vi "Get Class Referernce.vi"(8 "error in (no error)":errorcluster, 10 "ClassName":string, 11 "Application in":refnum<class "Application.lvclass">) -> (0 "error out":errorcluster, 3 "Application out":refnum<class "Application.lvclass">)   [LabVIEW 2019, in "Application.lvclass"]
doc: "Developed by Kevin Thompson\nkevin@thompsonengineering.net\n\nCopyright 2020\nThompson Engineering, LLC"
uses:
  Application.lvclass
panel:
  out "LabVIEW Object":refnum<class>
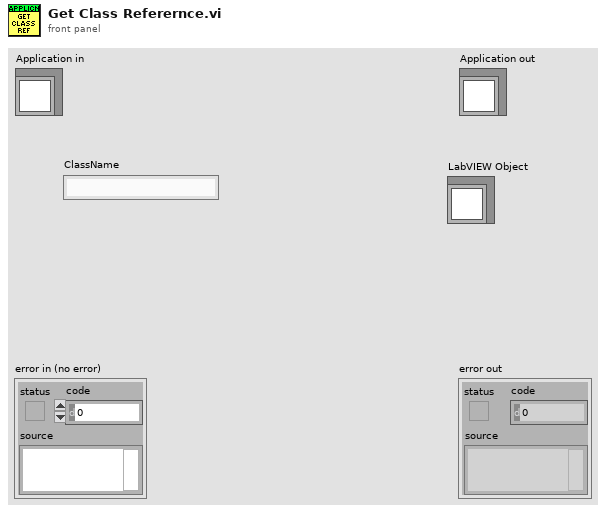
[diagram p1: front panel]
types:
  T1 = typedef "Application.lvclass/ObjData--cluster.ctl" = cluster{"Settings":T2, "Public Events":T3, "Dependency":T4, "ReadData-placeholder":T5, "VISA-placeholder":refnum<visa-resource-name>, "Subsys ClassRefs Dict":T6, "InverterWaveformsQ":T7, "RawDaqDataQ":T8}
  T2 = typedef "Application.lvclass/Settings--cluster.ctl" = cluster{"Simulation":bool}
  T3 = typedef "Application.lvclass/Public Events--cluster.ctl" = cluster{"Application.AsyncCmd Event":refnum<user-event>, "Application.AsyncMsg Event":refnum<user-event>, "stop process":refnum<user-event>}
  T4 = typedef "Application.lvclass/Dependency--cluster.ctl" = cluster{"Config":refnum<class "Config.lvclass">, "Main":refnum<class "Main.lvclass">, "ErrorHandler":refnum<class "ErrorHandler.lvclass">, "DAQ_Engine":refnum<class "DAQ_Engine.lvclass">, "Log_Engine":refnum<class "Log_Engine.lvclass">}
  T5 = typedef "Application.lvclass/Read Data--cluster.ctl" = cluster{"Data":dbl}
  T6 = typedef "TD Dynamic CVT DVR--ref.ctl" = refnum<data-value>
  T7 = typedef "InverterWaveforms--QRef.ctl" = refnum<queue>
  T8 = typedef "RawDAQDataQRef--cluster.ctl" = refnum<queue>
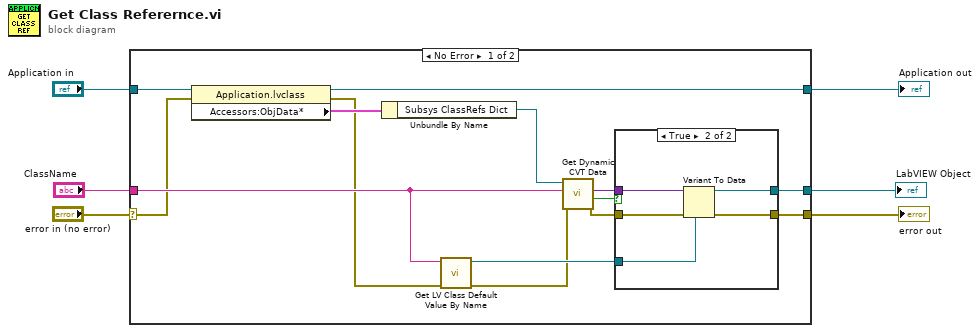
[diagram p0: block diagram]
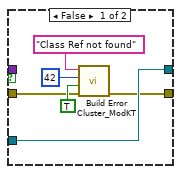
[diagram p2: hidden frame]
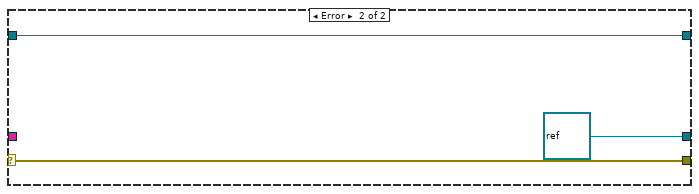
[diagram p3: hidden frame]
diagram:
  n1 = case shown="No Error" "error in (no error)" {
    selector: "error in (no error)" -> [w12 w34]
    tunnel: [w9 w34] -> w5
    tunnel: [w19 w33] -> w3
    tunnel: "Application in" -> [w20 w33]
    tunnel: "ClassName" -> [w14 _]
    tunnel: [w11 refnum<class> refnum ("object")] -> w1
    frame No Error {
      n2 = property class="Application.lvclass"(reference=w20, error in=w12) -> (reference out=w19:refnum<class "Application.lvclass">, error out=w13:errorcluster, "Accessors:ObjData*"=w18:T1)
      n3 = Unbundle By Name(w18) -> ("Subsys ClassRefs Dict"=w17:T6)
      n4 = call <vilib>:"Get LV Class Default Value By Name.vi"("error in (no error)"=w13, "class name"=w14) -> ("error out"=w10:errorcluster, "object"=w15:refnum<class>)  [unwired: 8 in]
      n5 = call <vilib>:"Get Dynamic CVT Data.vi"("error in (no error)"=w10, "DataName"=w14, "dCVT DVR"=w17) -> ("error out"=w7:errorcluster, "found"=w8:bool, "value"=w16:variant)  [unwired: 5 in, 1 out]
      n6 = case shown="True" w8 {
        tunnel: w16 -> [_ w31]
        tunnel: w15 -> [w26 w30]
        tunnel: [w26 w29] -> w11
        tunnel: [w25 w28] -> w9
        tunnel: w7 -> [w21 w27]
        frame False {
          n7 = call <vilib>:"Build Error Cluster_ModKT .vi"("Prepend String (\"\")"="Class Ref not found" ("Prepend String (\"\")"), "code"=42, "error? (F)"=TRUE, "error in (no error)"=w21) -> ("error out"=w25:errorcluster)  [unwired: 3 in, 1 out]
        }
        frame True {
          n8 = Variant To Data(error in=w27, type=w30, Variant=w31) -> (data=w29:refnum<class>, error out=w28:errorcluster)
        }
      }
    }
    frame Error {
    }
  }
  "error out" <- w5
  "Application out" <- w3
  "LabVIEW Object" <- w1
